vi "Creating a SubVI.vi"() -> ()   [LabVIEW 2010]
doc: "This VI demonstrates where to use subVIs to perform repeated calculations."
panel:
  in  "Function 3":cluster{"a":dbl, "b":dbl, "c":dbl, "d":dbl}
  in  "Function 2":cluster{"a":dbl, "b":dbl, "c":dbl, "d":dbl}
  in  "Function 1":cluster{"a":dbl, "b":dbl, "c":dbl, "d":dbl}
  out "XY Graph":cluster{i32[], dbl[]}[](graph)
  in  "Ending x value":i32=100
  in  "Starting x value":i32=-100
  # "ax^3+bx^2+cx+d"
  # "Domain"
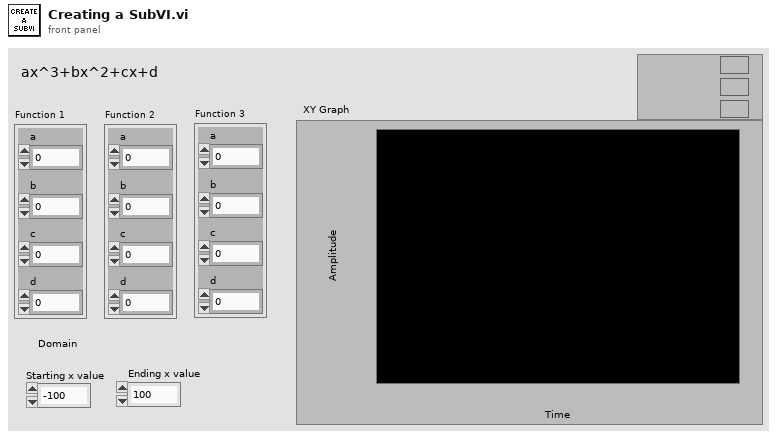
[diagram p1: front panel]
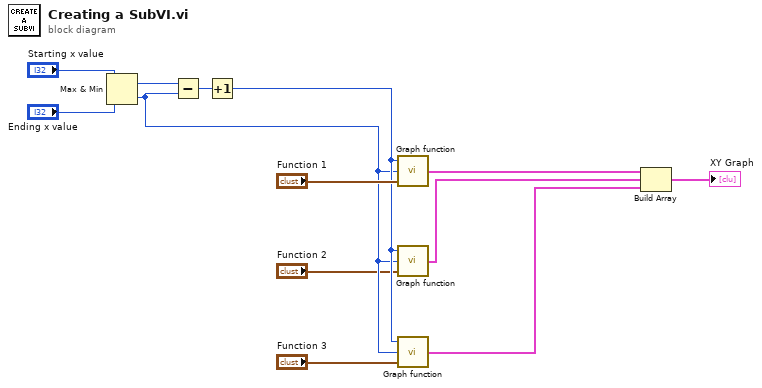
[diagram p0: block diagram]
diagram:
  n1 = Max & Min(x="Starting x value", y="Ending x value") -> (max(x,y)=w11:i32, min(x,y)=w5:i32)
  n2 = Subtract(x=w11, y=w5) -> (x-y=w10:i32)
  n3 = Increment(x=w10) -> (x+1=w6:i32)
  n4 = call "Graph function.vi"("Function 1"="Function 1", "Numeric 2"=w5, "Numeric"=w6) -> ("Cluster"=w9:cluster{i32[], dbl[]})
  n5 = call "Graph function.vi"("Function 1"="Function 2", "Numeric 2"=w5, "Numeric"=w6) -> ("Cluster"=w2:cluster{i32[], dbl[]})
  n6 = call "Graph function.vi"("Function 1"="Function 3", "Numeric 2"=w5, "Numeric"=w6) -> ("Cluster"=w1:cluster{i32[], dbl[]})
  n7 = Build Array(w9, w2, w1) -> (→"XY Graph":cluster{i32[], dbl[]}[])
